vi "Utility Write to Instrument.vi"(8 "error in (no error)":errorcluster, 10 "Write Buffer":string, 11 "VISA resource name":refnum<visa-resource-name>) -> (0 "error out":errorcluster, 2 "Read Buffer":string, 3 "VISA resource name out":refnum<visa-resource-name>)   [LabVIEW 2019, in "Quantum Composers 9000 Series.lvlib"]
doc: "This Utility VI is a wrapper which writes to the instrument and reads the response. This VI is intended to be used as a private VI and altering it could cause several public VI's to operate incorrectly."
uses:
  Quantum Composers 9000 Series.lvlib
  <vilib>/Utility/error.llb/DialogType.ctl
  Instance           2 35Saved   Utility Write to Instrument .vi
  Instance           1 35Saved   Utility Write to Instrument .vi
  Instance           3 35Saved   Utility Write to Instrument .vi
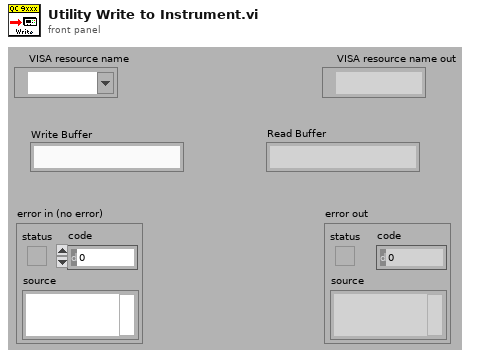
[diagram p1: front panel]
types:
  T1 = typedef "DialogType.ctl" = u16
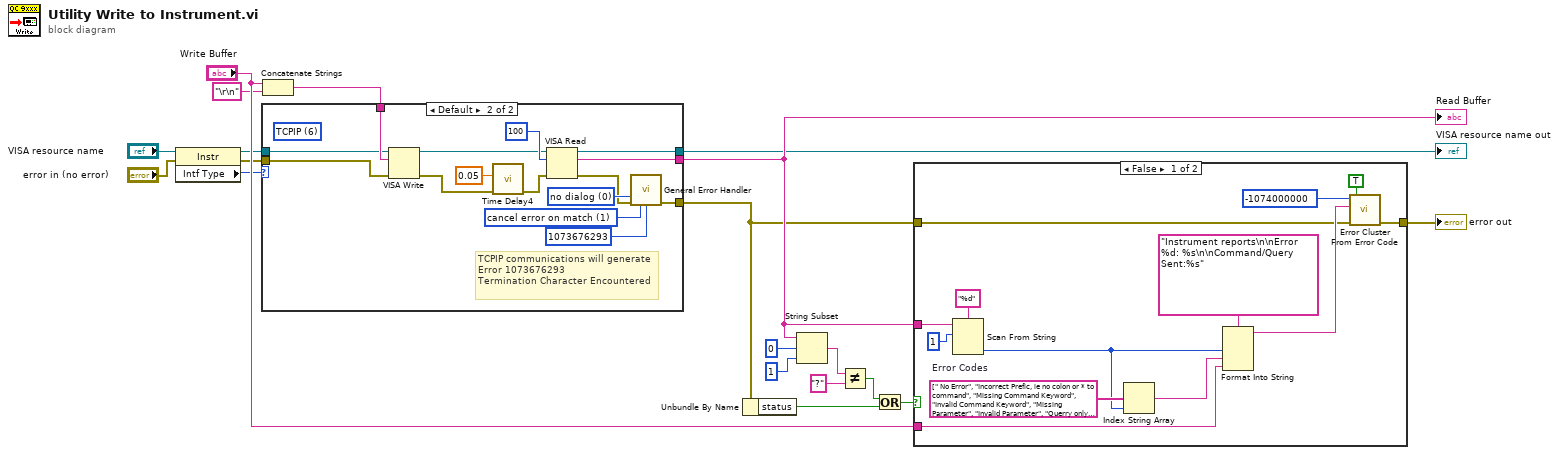
[diagram p0: block diagram]
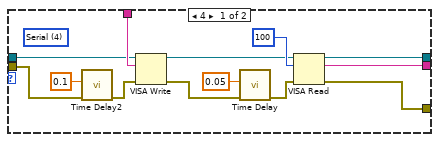
[diagram p2: hidden frame]
diagram:
  n1 = property class="Instr"(reference="VISA resource name", error in="error in (no error)") -> (reference out=w6:refnum<visa-resource-name>, error out=w5:errorcluster, "Intf Type"=w2:u16)
  n2 = Concatenate Strings("Write Buffer", "\r\n" ("string")) -> (w19:string)
  n3 = case shown="Default" w2 {
    tunnel: w19 -> [w32 w47]
    tunnel: [w30 w45] -> w14
    tunnel: [w29 w44] -> w9
    tunnel: [w28 w33] -> w1
    tunnel: w6 -> [w24 w41]
    tunnel: w5 -> [w23 w38]
    frame 4 {
      (unwired) u16 4 items=["GPIB"=1, "VXI"=2, "GPIB-VXI"=3, "Serial"=4, "PXI"=5, "TCPIP"=6, "USB"=7, "FireWire"=9] ("Interface Information:Interface Type")
      n4 = call "Time Delay2"("error in (no error)"=w23, "Delay Time (s)"=0.1) -> ("error out"=w25:errorcluster)  [unwired: 9 in]
      n5 = VISA Write(VISA resource name=w24, write buffer=w32, error in (no error)=w25) -> (VISA resource name out=w22:refnum<visa-resource-name>, error out=w26:errorcluster)  [unwired: 1 out]
      n6 = call "Time Delay"("error in (no error)"=w26, "Delay Time (s)"=0.05) -> ("error out"=w27:errorcluster)  [unwired: 9 in]
      n7 = VISA Read(VISA resource name=w22, byte count=u32 100, error in (no error)=w27) -> (VISA resource name out=w29:refnum<visa-resource-name>, read buffer=w30:string, error out=w28:errorcluster)  [unwired: 1 out]
    }
    frame Default {
      w37 = T1 0 items=["no dialog", "OK message", "continue or stop message", "OK message + warnings", "continue/stop + warnings"] ("type of dialog (OK msg:1)")
      (unwired) u16 6 items=["GPIB"=1, "VXI"=2, "GPIB-VXI"=3, "Serial"=4, "PXI"=5, "TCPIP"=6, "USB"=7, "FireWire"=9] ("Interface Information:Interface Type")
      w35 = 1 items=["no exception", "cancel error on match", "set error on match"] ("[exception action] (none:0)")
      # "TCPIP communications will generate\nError 1073676293\nTermination Character Encountered"
      n8 = VISA Write(VISA resource name=w41, write buffer=w47, error in (no error)=w38) -> (VISA resource name out=w40:refnum<visa-resource-name>, error out=w42:errorcluster)  [unwired: 1 out]
      n9 = call "Time Delay4"("error in (no error)"=w42, "Delay Time (s)"=0.05) -> ("error out"=w43:errorcluster)  [unwired: 9 in]
      n10 = VISA Read(VISA resource name=w40, byte count=u32 100, error in (no error)=w43) -> (VISA resource name out=w44:refnum<visa-resource-name>, read buffer=w45:string, error out=w34:errorcluster)  [unwired: 1 out]
      n11 = call <vilib>:"General Error Handler.vi"("type of dialog (OK msg:1)"=w37, "error in (no error)"=w34, "[exception action] (none:0)"=w35, "[exception code]"=1073676293) -> ("error out"=w33:errorcluster)  [unwired: 7 in, 4 out]
    }
  }
  "Read Buffer" <- w14
  "VISA resource name out" <- w9
  n12 = Unbundle By Name(w1) -> ("status"=w10:bool)
  n13 = String Subset(string=w14, offset (0)=0, length (rest)=1 ("length (rest)")) -> (substring=w11:string)
  n14 = Not Equal?(x=w11, y="?" ("x")) -> (x != y?=w13:bool)
  n15 = Or(x=w13, y=w10) -> (x .or. y?=w18:bool)
  n16 = case shown="False" w18 {
    tunnel: w14 -> [w59 _]
    tunnel: [w50 w61] -> w17
    tunnel: w1 -> [w48 w61]
    tunnel: "Write Buffer" -> [w54 _]
    frame False {
      w57 = string[] [" No Error", "Incorrect Prefic, ie no colon or * to command", "Missing Command Keyword", "Invalid Command Keyword", "Missing Parameter", "Invalid Parameter", "Querry only, command needs a question mark", "Invalid Query, command does not have a query form"]  # Error Codes
      n17 = Scan From String(format string="%d" ("Format String"), input string=w59, initial scan location=u32 1) -> (output 1=w56:i32)  [unwired: 2 in, 3 out]
      n18 = Index String Array(1:w56, 2:w57) -> (0:w55:string)  [unwired: 1 in]
      n19 = Format Into String(format string="Instrument reports\n\nError %d: %s\n\nCommand/Query Sent:%s" ("Source"), w56, w55, w54) -> (resulting string=w49:string)  [unwired: 2 in, 1 out]
      n20 = call <vilib>:"Error Cluster From Error Code.vi"("show call chain? (False)"=TRUE, "error in (no error)"=w48, "error message (\"\")"=w49, "error code (0)"=-1074000000 ("Code")) -> ("error out"=w50:errorcluster)  [unwired: 5 in]
    }
    frame True {
    }
  }
  "error out" <- w17
